vi "test metadata.vi"() -> ()   [LabVIEW 2013, in "Tiff reader.lvlib"]
doc: "Test metadata code."
uses:
  Tiff reader.lvlib
  <vilib>/vision/NI_Vision_Development_Module.lvlib
panel:
  out "Array":string[](array[string])
  out "OK? 3":bool=TRUE
  out "IFD locations":u32[](array[numeric])
  in  "Metadata string 4":string="Here's some daasdfta for youasdfa...asdfawefw"
  out "Metadata string 3":string
  out "Image 3":T1(plugin-control)
  out "OK? 2":bool=TRUE
  out "Metadata string 2":string
  out "OK?":bool=TRUE
  in  "Metadata string":string="Here's somwefwefwefawefawefe data for you..."
  out "path":path
  in  "file path (use dialog)":path=path "C:/Users/dmilkie/Desktop/junk.tif"
  in  "X":i32=100
  in  "Y":i32=100
  out "Image 2":T1(plugin-control)
  out "Image":T1(plugin-control)
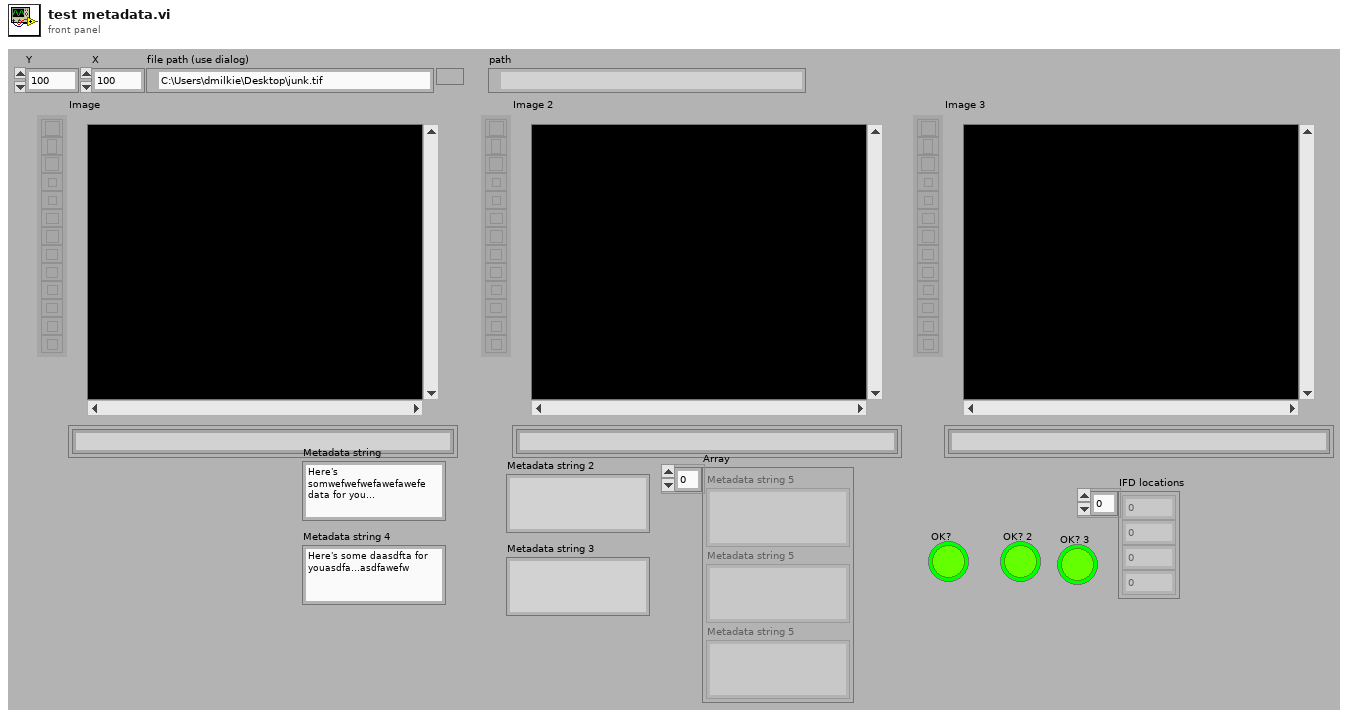
[diagram p1: front panel]
types:
  T1 = typedef "IMAQ Image.ctl" = refnum<image>
  T2 = typedef "Image Type" = u32
  T3 = enum16{"open", "replace", "create", "open or create", "replace or create", "replace or create with confirmation"}
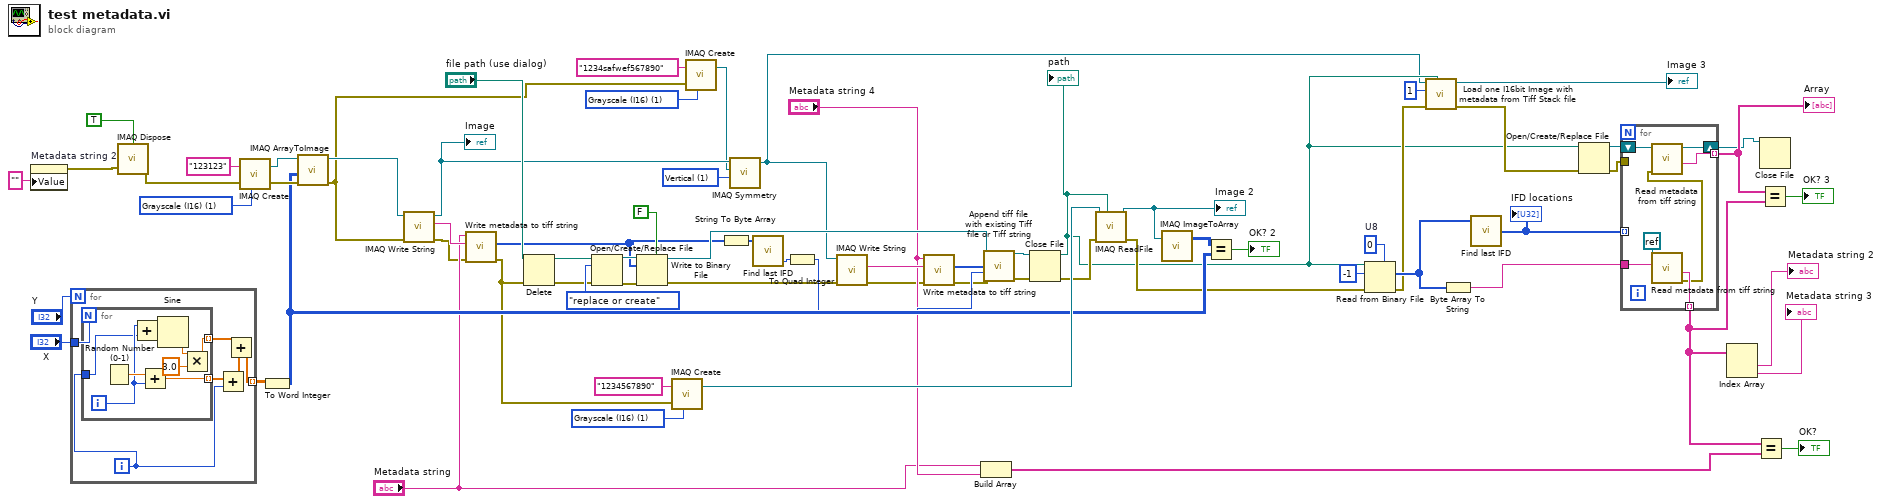
[diagram p0: block diagram]
diagram:
  w17 = u8 0  # U8
  w32 = T2 1 items=["Grayscale (U8)", "Grayscale (I16)", "Grayscale (SGL)", "Complex (CSG)", "RGB (U32)", "HSL (U32)", "RGB (U64)", "Grayscale (U16)"] ("Image Type")
  w49 = u32 1 items=["Horizontal", "Vertical", "Central", "1st Diagonal", "2nd Diagonal"] ("Type of Symmetry")
  w63 = T2 1 items=["Grayscale (U8)", "Grayscale (I16)", "Grayscale (SGL)", "Complex (CSG)", "RGB (U32)", "HSL (U32)", "RGB (U64)", "Grayscale (U16)"] ("Image Type")
  w71 = T2 1 items=["Grayscale (U8)", "Grayscale (I16)", "Grayscale (SGL)", "Complex (CSG)", "RGB (U32)", "HSL (U32)", "RGB (U64)", "Grayscale (U16)"] ("Image Type")
  n1 = property on="Metadata string 2" class="Str"("Value"="" ("Metadata string 2")) -> (error out=w51:errorcluster)  [unwired: 2 in, 1 out]
  n2 = for {
    N: "Y" -> [_]
    tunnel: [w74] -> w55 mode=indexing
    tunnel: "X" -> [w77]
    i -> [w73]
    n3 = for {
      N: w77 -> [_]
      tunnel: [w85] -> w78 mode=indexing
      tunnel: [w83] -> w76 mode=indexing
      tunnel: w73 -> [w79]
      i -> [w81]
      n4 = Random Number (0-1)() -> (number: 0 to 1=w86:dbl)
      n5 = Add(x=w81, y=w79) -> (x+y=w80:i32)
      n6 = Add(x=w86, y=w81) -> (x+y=w85:dbl)
      n7 = Sine(x=w80) -> (sin(x)=w84:dbl)
      n8 = Multiply(x=w84, y=3.0) -> (x*y=w83:dbl)
    }
    n9 = Add(x=w78, y=w73) -> (x+y=w75:dbl[])
    n10 = Add(x=w76, y=w75) -> (x+y=w74:dbl[])
  }
  n11 = call "IMAQ Dispose"("All Images? (No)"=TRUE, "error in (no error)"=w51) -> ("error out"=w59:errorcluster)  [unwired: 1 in, 3 out]
  n12 = call "IMAQ Create"("Image Name"="123123", "Image Type"=w71, "error in (no error)"=w59) -> ("New Image"=w70:T1, "error out"=w60:errorcluster)  [unwired: 1 in, 1 out]
  n13 = To Word Integer(number=w55) -> (16bit integer=w52:i16[][])
  n14 = call "IMAQ ArrayToImage"("error in (no error)"=w60, "Image Pixels (I16)"=w52, "Image"=w70) -> ("error out"=w23:errorcluster, "Image Out"=w57:T1)  [unwired: 3 in, 4 out]
  n15 = call-poly "IMAQ Write String"("error in (no error)"=w23, "Image"=w57) -> ("error out"=w2:errorcluster, "FileString"=w21:string, "Image Out (duplicate)"=w25:T1)  [unwired: 2 in, 5 out]
  "Image" <- w25
  n16 = call "Write metadata to tiff string.vi"("error in"=w2, "Tiff image (unsigned byte array)"=w21, "Metadata string\n(must be at least 5 char long)"="Metadata string") -> ("error out"=w1:errorcluster, "Tiff file out (unsigned byte array)"=w22:u8[])  [unwired: 1 in, 6 out]
  n17 = Delete(path (use dialog)="file path (use dialog)", error in=w1) -> (deleted path=w27:path, error out=w28:errorcluster)  [unwired: 4 out]
  n18 = Open/Create/Replace File(file path (use dialog)=w27, error in=w28, operation (0:open)=T3."replace or create") -> (refnum out=w66:refnum<file>, error out=w65:errorcluster)  [unwired: 4 out]
  n19 = Write to Binary File(file (use dialog)=w66, data=w22, error in=w65, 5:FALSE ("prepend array or string size? (T)")) -> (refnum out=w46:refnum<file>, error out=w44:errorcluster)  [unwired: 3 out]
  n20 = call "IMAQ Create"("Image Name"="1234567890", "Image Type"=w63, "error in (no error)"=w1) -> ("New Image"=w61:T1)  [unwired: 1 in, 2 out]
  n21 = call "IMAQ Create"("Image Name"="1234safwef567890", "Image Type"=w32, "error in (no error)"=w23) -> ("New Image"=w24:T1)  [unwired: 1 in, 2 out]
  n22 = String To Byte Array(string=w22) -> (unsigned byte array=w48:u8[])
  n23 = call "IMAQ Symmetry"("Type of Symmetry"=w49, "Image Dst"=w24, "Image Src"=w25) -> ("Image Dst Out"=w7:T1)  [unwired: 1 in, 2 out]
  n24 = call "Find last IFD.vi"("TIFF Data in"=w48) -> ("Location in byte stream of last IFD pointer.  This\nis the word to change if you are adding another page\nto the file."=w47:i32)  [unwired: 4 out]
  n25 = To Quad Integer(1:w47) -> (0:w45:i64)
  n26 = call-poly "IMAQ Write String"("error in (no error)"=w44, "Image"=w7) -> ("error out"=w3:errorcluster, "FileString"=w40:string)  [unwired: 2 in, 6 out]
  n27 = call "Write metadata to tiff string.vi"("error in"=w3, "Tiff image (unsigned byte array)"=w40, "Metadata string\n(must be at least 5 char long)"="Metadata string 4") -> ("error out"=w4:errorcluster, "Tiff file out (unsigned byte array)"=w39:u8[])  [unwired: 1 in, 6 out]
  n28 = Build Array("Metadata string", "Metadata string 4") -> (w34:string[])
  n29 = call "Append tiff file with existing Tiff file or Tiff string.vi"("Existing Tiff File (A) refnum"=w46, "Tiff file (B)\n (unsigned byte array)"=w39, "Location in existing file of\nit's last page's \n\"next IFD pointer\""=w45, "error in"=w4) -> ("File refnum out"=w43:refnum<file>, "error out"=w42:errorcluster)  [unwired: 3 in, 7 out]
  n30 = Close File(refnum=w43, error in=w42) -> (path=w8:path, error out=w41:errorcluster)
  "path" <- w8
  n31 = call "IMAQ ReadFile"("File Path"=w8, "error in (no error)"=w41, "Image"=w61) -> ("error out"=w38:errorcluster, "Image Out"=w56:T1)  [unwired: 2 in, 5 out]
  "Image 2" <- w56
  n32 = call "IMAQ ImageToArray"("Image"=w56) -> ("Image Pixels (I16)"=w53:i16[][])  [unwired: 2 in, 5 out]
  n33 = Equal?(x=w53, y=w52) -> (x = y?=→"OK? 2":bool)
  n34 = Read from Binary File(5:w17, 8:w38, 10:-1 ("count (1)"), 11:w8) -> (0:w16:errorcluster, 2:w19:u8[])  [unwired: 4 out]
  n35 = call "Load one I16bit Image with metadata from Tiff Stack file.vi"("path to TIFF file"=w8, "error in"=w16, "Index of image\n to read"=1 ("Index of image to read"), "I16 Image"=w7) -> ("error out"=w15:errorcluster, "I16 Image dup"=→"Image 3":T1)  [unwired: 6 out]
  n36 = Byte Array To String(unsigned byte array=w19) -> (string=w18:string)
  n37 = call "Find last IFD.vi"("TIFF Data in"=w19) -> ("IFD locations"=w36:u32[])  [unwired: 4 out]
  "IFD locations" <- w36
  n38 = Open/Create/Replace File(file path (use dialog)=w8, error in=w15) -> (refnum out=w14:refnum<file>, error out=w5:errorcluster)  [unwired: 5 out]
  n39 = for {
    tunnel: w18 -> [w88]
    tunnel: w36 -> [_] mode=indexing
    tunnel: [w93] -> w11 mode=indexing
    tunnel: [w92] -> w12 mode=indexing
    shift-right: [w89] -> w10
    shift-left: w14 -> [w90]
    tunnel: w5 -> [_]
    n40 = call "Read metadata from tiff string.vi"(10:"Tiff image stack"=w88, 11:"Tiff image stack"=refnum<k0> refnum) -> ("error out"=w91:errorcluster, "Metadata string"=w93:string)  [unwired: 2 in, 6 out]
    n41 = call "Read metadata from tiff string.vi"("error in"=w91, "Tiff image stack"=w90) -> ("Metadata string"=w92:string, "Tiff image stack dup"=w89:refnum<file>)  [unwired: 2 in, 6 out]
  }
  "Array" <- w12
  n42 = Index Array(array=w11) -> (element #1=→"Metadata string 2":string, element #2=→"Metadata string 3":string)  [unwired: 2 in]
  n43 = Equal?(x=w11, y=w34) -> (x = y?=→"OK?":bool)
  n44 = Close File(refnum=w10) -> ()  [unwired: 1 in, 2 out]
  n45 = Equal?(x=w12, y=w11) -> (x = y?=→"OK? 3":bool)
